vi "Read error correction.vi"(8 "error in (no error)":errorcluster, 9 "Recieve data":string, 10 "Sent command header":string, 11 "connection ID":refnum<k5>) -> (0 "error out":errorcluster, 1 "TCP Error":bool, 2 "Data Error":bool, 3 "connection ID out":refnum<k5>)   [LabVIEW 2019, in "LifterTCP.lvclass"]
uses:
  LifterTCP.lvclass
panel:
  out "Recieved header":string
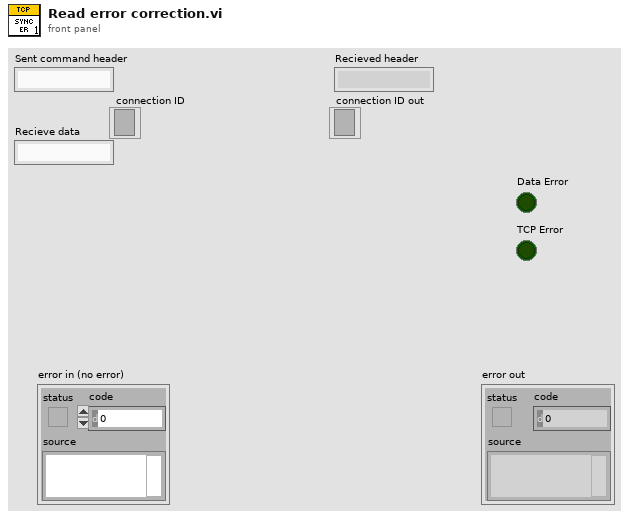
[diagram p1: front panel]
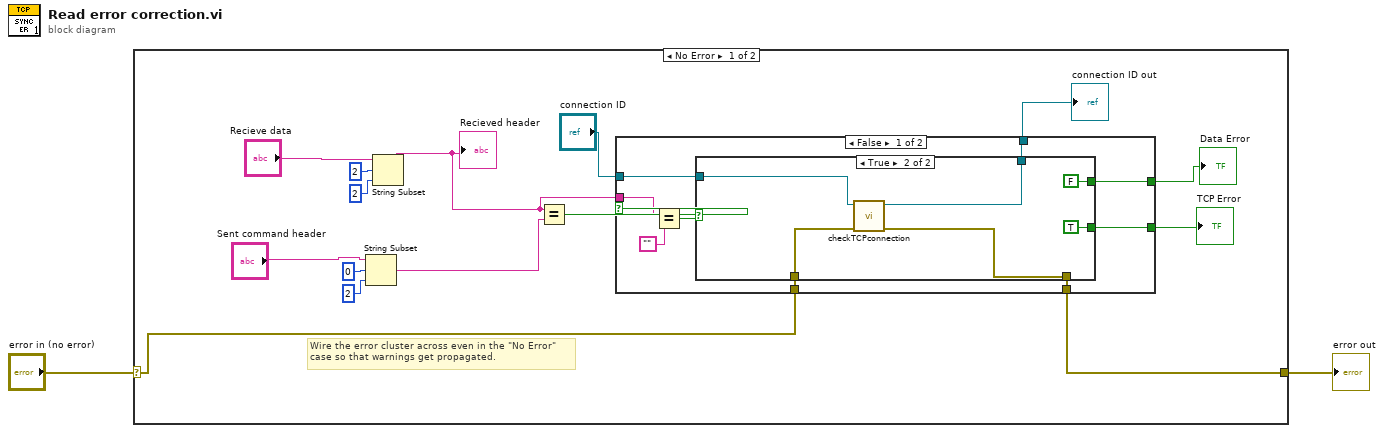
[diagram p0: block diagram]
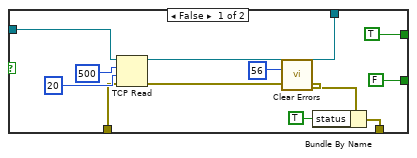
[diagram p2: hidden frame]
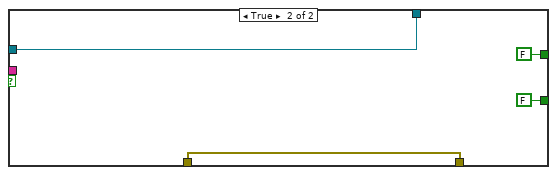
[diagram p3: hidden frame]
diagram:
  n1 = case shown="No Error" "error in (no error)" {
    selector: "error in (no error)" -> [w13 w49]
    tunnel: [w12 w49] -> w1
    frame No Error {
      # "Wire the error cluster across even in the \"No Error\"\ncase so that warnings get propagated."
      n2 = String Subset(string="Sent command header", offset (0)=0, length (rest)=2 ("length (rest)")) -> (substring=w6:string)
      n3 = String Subset(string="Recieve data", offset (0)=2, length (rest)=2 ("length (rest)")) -> (substring=w5:string)
      "Recieved header" <- w5
      n4 = Equal?(x=w5, y=w6) -> (x = y?=w14:bool)
      n5 = case shown="False" w14 {
        tunnel: w13 -> [w26 w48]
        tunnel: [w23 w48] -> w12
        tunnel: "connection ID" -> [w25 w47]
        tunnel: [w24 w47] -> w10
        tunnel: w5 -> [w20 _]
        tunnel: [w19 FALSE ("TCP Error")] -> w4
        tunnel: [w18 FALSE ("Data Error")] -> w3
        frame False {
          n6 = Equal?(x=w20, y="") -> (x = y?=w22:bool)
          n7 = case shown="True" w22 {
            tunnel: w26 -> [w36 w42]
            tunnel: w25 -> [w35 w44]
            tunnel: [w34 w43] -> w24
            tunnel: [w30 w41] -> w23
            tunnel: [FALSE ("TCP Error") TRUE ("TCP Error")] -> w19
            tunnel: [TRUE ("Data Error") FALSE ("Data Error")] -> w18
            frame False {
              n8 = TCP Read(connection ID=w35, bytes to read=500, error in (no error)=w36, 9:20 ("timeout ms (25000)")) -> (connection ID out=w34:refnum<k5>, error out=w32:errorcluster)  [unwired: 1 in, 1 out]
              n9 = call <vilib>:"Clear Errors.vi"("error in (no error)"=w32, "specific error code to clear (0: all)"=56) -> ("error out"=w31:errorcluster)  [unwired: 4 in, 1 out]
              n10 = Bundle By Name(cluster=w31, "status"=TRUE) -> (w30:errorcluster)
            }
            frame True {
              n11 = call "checkTCPconnection.vi"("error in (no error)"=w42, "connection ID"=w44) -> ("error out"=w41:errorcluster, "connection IDout"=w43:refnum<k5>)  [unwired: 8 in]
            }
          }
        }
        frame True {
        }
      }
      "connection ID out" <- w10
      "Data Error" <- w3
      "TCP Error" <- w4
    }
    frame Error {
    }
  }
  "error out" <- w1
